vi "PWM CAP Stop.vi"(10 "Channel":u8, 11 "DevHandle":i32) -> (3 "function return":i32)   [LabVIEW 2010, in "usb2pwm.lvlib"]
doc: "int WINAPI PWM_CAP_Stop(int DevHandle, unsigned char Channel);"
uses:
  usb2pwm.lvlib
  USB2XXX/trunk/USB2XXX/USB2XXX/vs2019/Release/USB2XXX.dll
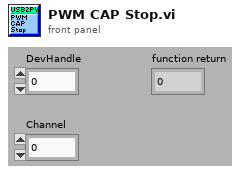
[diagram p1: front panel]
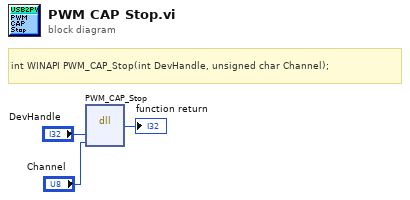
[diagram p0: block diagram]
diagram:
  # "int WINAPI PWM_CAP_Stop(int DevHandle, unsigned char Channel);"
  n1 = dll-call lib="E:/Projects/USB2XXX/trunk/USB2XXX/USB2XXX/vs2019/Release/USB2XXX.*" fn="PWM_CAP_Stop"("DevHandle"="DevHandle", "Channel"="Channel") -> (→"function return":i32)  [unwired: 5 in, 2 out]
